vi "adam-sample-analog.vi"(7 "Analog Data":T1, 8 "error in (no error)":errorcluster, 11 "VISA Refnum in":refnum<visa-resource-name>) -> (0 "error out":errorcluster, 1 "status":string, 2 "read buffer":string, 3 "VISA Refnum out":refnum<visa-resource-name>, 4 "acknowledge char":string, 5 "Analog Data Out":T1)   [LabVIEW 2024]
uses:
  controls/depreciated/analog-data-cluster.ctl
panel:
  in  "chassis slot":u8=2
  in  "ADAM-5000: Chassis ID":u8=1
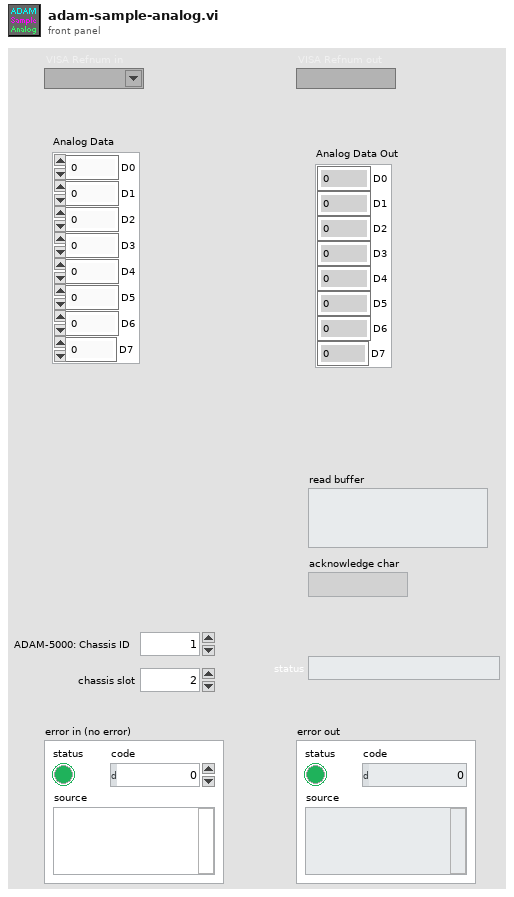
[diagram p1: front panel]
types:
  T1 = typedef "analog-data-cluster.ctl" = cluster{"D0":dbl, "D1":dbl, "D2":dbl, "D3":dbl, "D4":dbl, "D5":dbl, "D6":dbl, "D7":dbl}
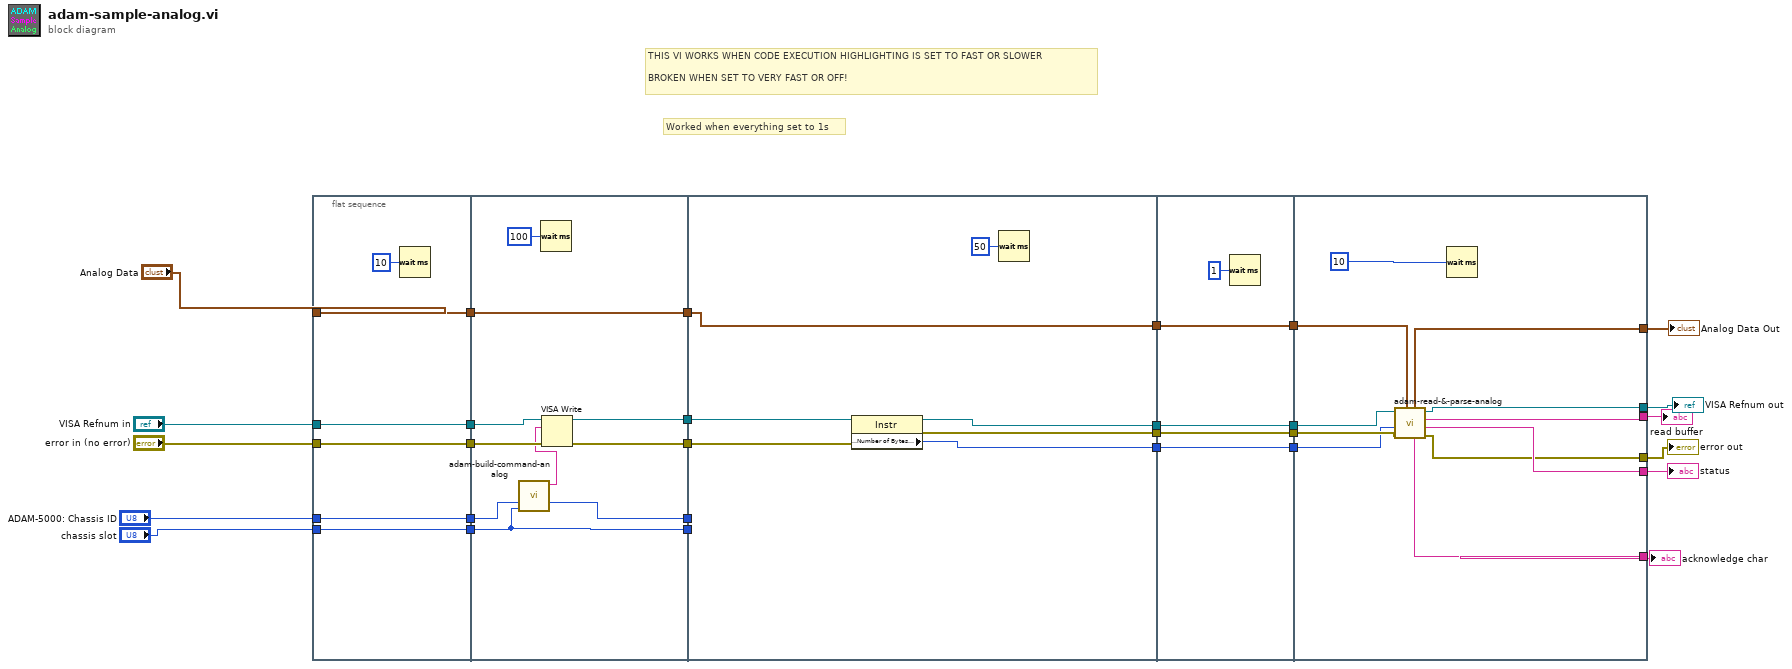
[diagram p0: block diagram]
diagram:
  # "Worked when everything set to 1s"
  # "THIS VI WORKS WHEN CODE EXECUTION HIGHLIGHTING IS SET TO FAST OR SLOWER\n\nBROKEN WHEN SET TO VERY FAST OR OFF!"
  n1 = flat-sequence {
    tunnel: "Analog Data" -> [w31]
    tunnel: "ADAM-5000: Chassis ID" -> [w32]
    tunnel: "chassis slot" -> [w33]
    tunnel: "VISA Refnum in" -> [w34]
    tunnel: "error in (no error)" -> [w35]
    tunnel: [w35] -> w9
    tunnel: [w34] -> w8
    tunnel: [w33] -> w7
    tunnel: [w32] -> w6
    tunnel: [w31] -> w5
    tunnel: [w38] -> w12
    tunnel: [w37] -> w11
    tunnel: [w43] -> w10
    tunnel: w9 -> [w44]
    tunnel: w8 -> [w41]
    tunnel: w7 -> [w38]
    tunnel: w6 -> [w37]
    tunnel: w5 -> [w43]
    tunnel: [w42] -> w4
    tunnel: [w40] -> w3
    tunnel: [w51] -> w29
    tunnel: [w50] -> w28
    tunnel: [w49] -> w27
    tunnel: [w48] -> w13
    tunnel: w12 -> [_]
    tunnel: w11 -> [_]
    tunnel: w10 -> [w48]
    tunnel: w4 -> [w46]
    tunnel: w3 -> [w45]
    tunnel: w29 -> [w56]
    tunnel: w28 -> [w55]
    tunnel: w27 -> [w54]
    tunnel: [w56] -> w26
    tunnel: [w55] -> w25
    tunnel: [w54] -> w24
    tunnel: [w52] -> w14
    tunnel: w13 -> [w52]
    tunnel: w26 -> [w65]
    tunnel: w25 -> [w66]
    tunnel: w24 -> [w64]
    tunnel: [w60] -> w19
    tunnel: [w61] -> w18
    tunnel: [w62] -> w15
    tunnel: [w63] -> w17
    tunnel: [w59] -> w16
    tunnel: w14 -> [w58]
    tunnel: [w57] -> w1
    frame #0 {
      n2 = Wait (ms)(milliseconds to wait=u32 10) -> ()  [unwired: 1 out]
    }
    frame #1 {
      n3 = call "adam-build-command-analog.vi"("chassis slot"=w38, "ADAM-5000: Chassis ID"=w37) -> ("Command Out"=w36:string)  [unwired: 9 in]
      n4 = Wait (ms)(milliseconds to wait=u32 100) -> ()  [unwired: 1 out]
      n5 = VISA Write(VISA resource name=w41, write buffer=w36, error in (no error)=w44) -> (VISA resource name out=w40:refnum<visa-resource-name>, error out=w42:errorcluster)  [unwired: 1 out]
    }
    frame #2 {
      n6 = property class="Instr"(reference=w45, error in=w46) -> (reference out=w50:refnum<visa-resource-name>, error out=w51:errorcluster, "Serial Settings:Number of Bytes at Serial Port"=w49:u32)
      n7 = Wait (ms)(milliseconds to wait=u32 50) -> ()  [unwired: 1 out]
    }
    frame #3 {
      n8 = Wait (ms)(milliseconds to wait=u32 1) -> ()  [unwired: 1 out]
    }
    frame #4 {
      n9 = call "adam-read-&-parse-analog.vi"("Analog Data"=w58, "error in (no error)"=w65, "Bytes at Port"=w64, "VISA Refnum in"=w66) -> ("error out"=w60:errorcluster, "status  out"=w61:string, "read buffer"=w62:string, "VISA Refnum out"=w63:refnum<visa-resource-name>, "acknowledge char"=w59:string, "Analog Data Out"=w57:T1)  [unwired: 2 in]
      n10 = Wait (ms)(milliseconds to wait=u32 10) -> ()  [unwired: 1 out]
    }
  }
  "status" <- w18
  "error out" <- w19
  "VISA Refnum out" <- w17
  "read buffer" <- w15
  "acknowledge char" <- w16
  "Analog Data Out" <- w1
